vi "Write Color.vi"(8 "error in (no error)":errorcluster, 10 "Color":u32(colorbox), 11 "Splitter in":refnum<class "Splitter.lvclass">) -> (0 "error out":errorcluster, 3 "Splitter out":refnum<class "Splitter.lvclass">)   [LabVIEW 2015, in "Splitter.lvclass"]
uses:
  Splitter.lvclass
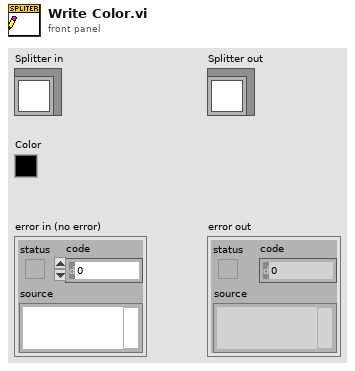
[diagram p1: front panel]
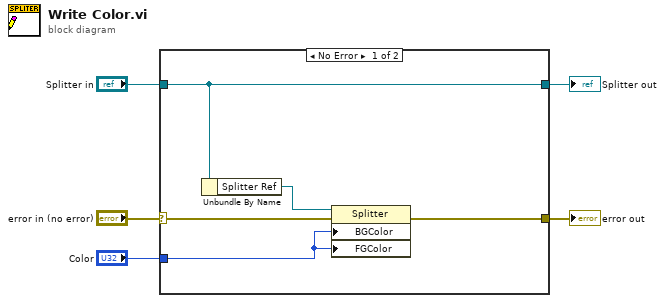
[diagram p0: block diagram]
diagram:
  n1 = case shown="No Error" "error in (no error)" {
    selector: "error in (no error)" -> [w10 w11]
    tunnel: [w9 w11] -> w4
    tunnel: [w8 w12] -> w2
    tunnel: "Splitter in" -> [w8 w12]
    tunnel: "Color" -> [w6 _]
    frame No Error {
      n2 = Unbundle By Name(w8) -> ("Splitter Ref"=w7:refnum<vi>)
      n3 = property class="Splitter"(reference=w7, error in=w10, "BGColor"=w6, "FGColor"=w6) -> (error out=w9:errorcluster)  [unwired: 1 out]
    }
    frame Error {
    }
  }
  "error out" <- w4
  "Splitter out" <- w2
